vi "Default Group Name.vi"(0 "group name in":string) -> (4 "group name out":string)   [LabVIEW 2021, in "InstrumentStudio Plug-In Editor.lvlib"]
uses:
  InstrumentStudio Plug-In Editor.lvlib
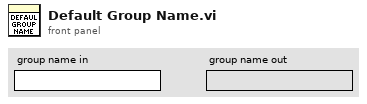
[diagram p1: front panel]
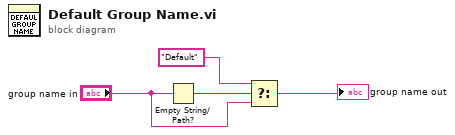
[diagram p0: block diagram]
diagram:
  n1 = Empty String/Path?(string/path="group name in") -> (empty?=w2:bool)
  n2 = Select(t="Default", s=w2, f="group name in") -> (s? t:f=→"group name out":string)
